vi "Dispose.vi"(8 "error in (no error)":errorcluster, 11 "Class 1 in":refnum<class "Freetype Drawer.lvclass">) -> (0 "error out":errorcluster)   [LabVIEW 2023, in "Freetype Drawer.lvlib" / "Freetype Drawer.lvclass"]
uses:
  Freetype Drawer.lvclass
  Freetype Drawer.lvclass/Freetype Drawer.ctl
  Freetype Drawer.lvlib
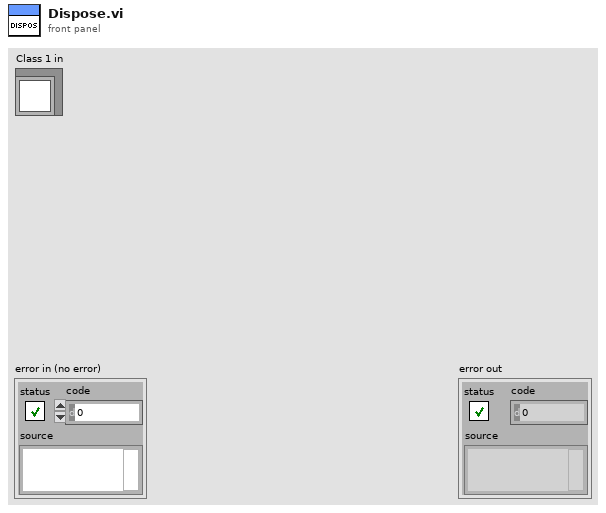
[diagram p1: front panel]
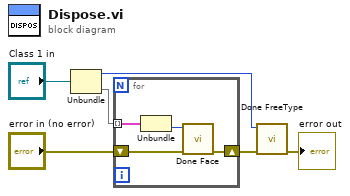
[diagram p0: block diagram]
diagram:
  n1 = Unbundle("Class 1 in") -> (w5:i64, w3:map{string, i64})  [unwired: 1 out]
  n2 = for {
    tunnel: w3 -> [w10] mode=indexing
    shift-right: [w7] -> w1
    shift-left: "error in (no error)" -> [w9]
    n3 = Unbundle(w10) -> ("face ref"=w8:i64)  [unwired: 1 out]
    n4 = call "Done Face.vi"("error in (no error)"=w9, "face in"=w8) -> ("error out"=w7:errorcluster)  [unwired: 9 in]
  }
  n5 = call "Done FreeType.vi"("error in (no error)"=w1, "library in"=w5) -> ("error out"=→"error out":errorcluster)  [unwired: 9 in]
